vi "initialize_dcs.vi"(8 "error in (no error)":errorcluster) -> (0 "error out":errorcluster, 2 "Dust Spot Array":T1[](array[typedef]), 3 "Dust Point Array":T2[](array[typedef]))   [LabVIEW 2012]
uses:
  dcs points.ctl
  dcs_spot.ctl
  <vilib>/addons/database/Connection.llb/Conn Execute.vi
  <vilib>/addons/database/Recordset.llb/Rec Fetch Recordset Data (R).vi
  <vilib>/addons/database/Recordset.llb/Rec Destroy - Connection.vi
  <vilib>/addons/database/_DB Variant To Data/Database Variant To Data.xnode
  <vilib>/addons/database/NI_Database_API.lvlib
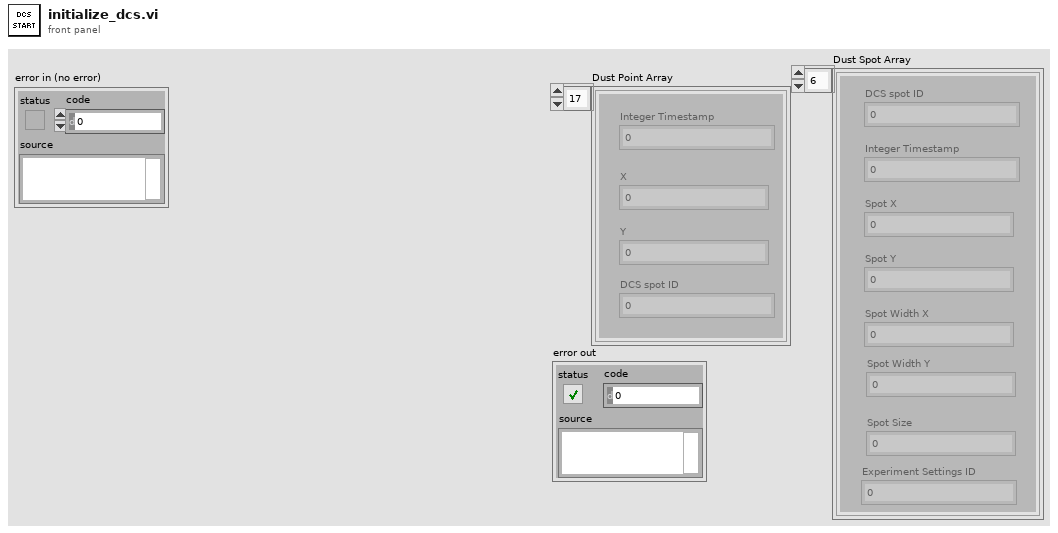
[diagram p1: front panel]
types:
  T1 = typedef "dcs_spot.ctl" = cluster{"DCS spot ID":i32, "Integer Timestamp":i64, "Spot X":dbl, "Spot Y":dbl, "Spot Width X":dbl, "Spot Width Y":dbl, "Spot Size":i32, "Experiment Settings ID":i32}
  T2 = typedef "dcs points.ctl" = cluster{"Integer Timestamp":i64, "X":dbl, "Y":dbl, "DCS spot ID":i32}
  T3 = typedef "NI_Database_API.lvlib/Conn ObjectReference.ctl" = refnum<k1>
  T4 = typedef "NI_Database_API.lvlib/Rec ObjectReference.ctl" = refnum<k1>
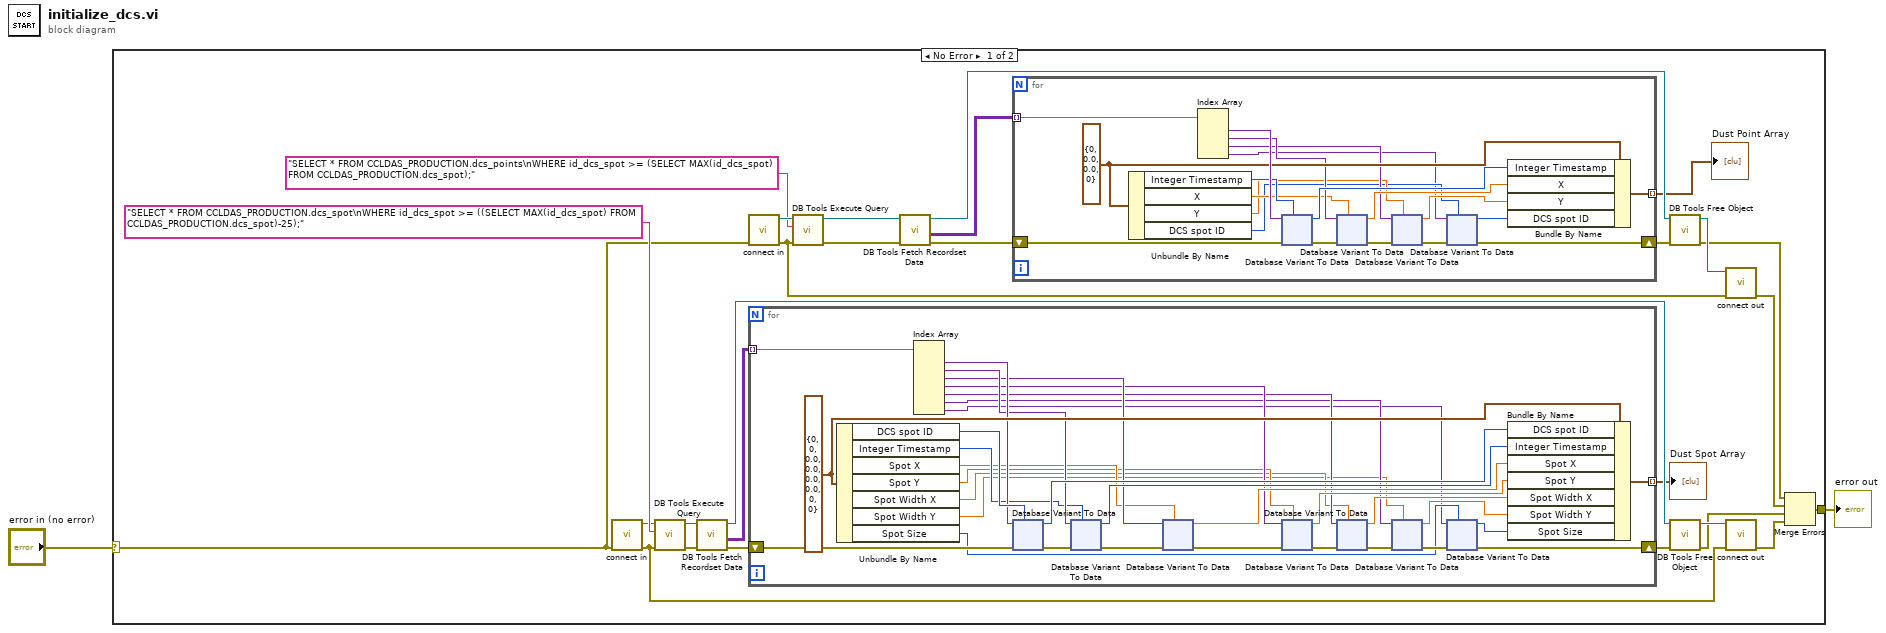
[diagram p0: block diagram]
diagram:
  n1 = case shown="No Error" "error in (no error)" {
    selector: "error in (no error)" -> [w21 w435]
    tunnel: [w3 w435] -> w1
    frame No Error {
      n2 = call "connect in.vi"("error in (no error)"=w21) -> ("error out"=w19:errorcluster, "Database Connection"=w20:T3)  [unwired: 6 in, 1 out]
      n3 = call-poly <vilib>:"DB Tools Execute Query.vi"("error in (no error)"=w19, "SQL query"="SELECT * FROM CCLDAS_PRODUCTION.dcs_spot\nWHERE id_dcs_spot >= ((SELECT MAX(id_dcs_spot) FROM CCLDAS_PRODUCTION.dcs_spot)-25);", "connection reference"=w20) -> ("error out"=w27:errorcluster, "recordset reference"=w28:T4)  [unwired: 5 in]
      n4 = call-poly <vilib>:"DB Tools Fetch Recordset Data.vi"("error in (no error)"=w27, "recordset reference"=w28) -> ("error out"=w8:errorcluster, "recordset data"=w9:variant[][], "recordset reference out"=w22:T4)  [unwired: 3 in]
      n5 = call "connect in.vi"("error in (no error)"=w21) -> ("error out"=w17:errorcluster, "Database Connection"=w26:T3)  [unwired: 6 in, 1 out]
      n6 = for {
        tunnel: w9 -> [w210] mode=indexing
        shift-right: [w182] -> w7
        shift-left: w8 -> [w207]
        tunnel: [w209] -> w4 mode=indexing
        w208 = T1 {"DCS spot ID"=0, "Integer Timestamp"=0, "Spot X"=0.0, "Spot Y"=0.0, "Spot Width X"=0.0, "Spot Width Y"=0.0, "Spot Size"=0, "Experiment Settings ID"=0} ("DCS spot")
        n7 = Unbundle By Name(w208) -> ("DCS spot ID"=w206:i32, "Integer Timestamp"=w201:i64, "Spot X"=w198:dbl, "Spot Y"=w193:dbl, "Spot Width X"=w189:dbl, "Spot Width Y"=w185:dbl, "Spot Size"=w180:i32)
        n8 = Index Array(array=w210) -> (element #1=w205:variant, element #2=w202:variant, element #3=w199:variant, element #4=w194:variant, element #5=w190:variant, element #6=w186:variant, element #7=w179:variant)  [unwired: 7 in]
        n9 = xnode "Database Variant To Data"("database variant"=w205, "error in (no error)"=w207, "type"=w206) -> ("data"=w204:i32, "error out"=w203:errorcluster)
        n10 = xnode "Database Variant To Data"("database variant"=w202, "error in (no error)"=w203, "type"=w201) -> ("data"=w200:i64, "error out"=w196:errorcluster)
        n11 = xnode "Database Variant To Data"("database variant"=w199, "error in (no error)"=w196, "type"=w198) -> ("data"=w197:dbl, "error out"=w195:errorcluster)
        n12 = xnode "Database Variant To Data"("database variant"=w194, "error in (no error)"=w195, "type"=w193) -> ("data"=w192:dbl, "error out"=w191:errorcluster)
        n13 = xnode "Database Variant To Data"("database variant"=w190, "error in (no error)"=w191, "type"=w189) -> ("data"=w188:dbl, "error out"=w187:errorcluster)
        n14 = xnode "Database Variant To Data"("database variant"=w186, "error in (no error)"=w187, "type"=w185) -> ("data"=w184:dbl, "error out"=w183:errorcluster)
        n15 = xnode "Database Variant To Data"("database variant"=w179, "error in (no error)"=w183, "type"=w180) -> ("data"=w181:i32, "error out"=w182:errorcluster)
        n16 = Bundle By Name(cluster=w208, "DCS spot ID"=w204, "Integer Timestamp"=w200, "Spot X"=w197, "Spot Y"=w192, "Spot Width X"=w188, "Spot Width Y"=w184, "Spot Size"=w181) -> (w209:T1)
      }
      "Dust Spot Array" <- w4
      n17 = call-poly <vilib>:"DB Tools Execute Query.vi"("error in (no error)"=w17, "SQL query"="SELECT * FROM CCLDAS_PRODUCTION.dcs_points\nWHERE id_dcs_spot >= (SELECT MAX(id_dcs_spot) FROM CCLDAS_PRODUCTION.dcs_spot);" ("format string"), "connection reference"=w26) -> ("error out"=w29:errorcluster, "recordset reference"=w30:T4)  [unwired: 5 in]
      n18 = call-poly <vilib>:"DB Tools Fetch Recordset Data.vi"("error in (no error)"=w29, "recordset reference"=w30) -> ("error out"=w10:errorcluster, "recordset data"=w11:variant[][], "recordset reference out"=w23:T4)  [unwired: 3 in]
      n19 = for {
        tunnel: w11 -> [w50] mode=indexing
        shift-right: [w37] -> w6
        shift-left: w10 -> [w44]
        tunnel: [w49] -> w5 mode=indexing
        w47 = T2 {"Integer Timestamp"=0, "X"=0.0, "Y"=0.0, "DCS spot ID"=0} ("DCS points")
        n20 = Unbundle By Name(w47) -> ("Integer Timestamp"=w46:i64, "X"=w41:dbl, "Y"=w35:dbl, "DCS spot ID"=w32:i32)
        n21 = Index Array(array=w50) -> (element #1=w48:variant, element #2=w42:variant, element #3=w36:variant, element #4=w31:variant)  [unwired: 4 in]
        n22 = xnode "Database Variant To Data"("database variant"=w48, "error in (no error)"=w44, "type"=w46) -> ("data"=w45:i64, "error out"=w43:errorcluster)
        n23 = xnode "Database Variant To Data"("database variant"=w42, "error in (no error)"=w43, "type"=w41) -> ("data"=w40:dbl, "error out"=w39:errorcluster)
        n24 = xnode "Database Variant To Data"("database variant"=w36, "error in (no error)"=w39, "type"=w35) -> ("data"=w34:dbl, "error out"=w38:errorcluster)
        n25 = xnode "Database Variant To Data"("database variant"=w31, "error in (no error)"=w38, "type"=w32) -> ("data"=w33:i32, "error out"=w37:errorcluster)
        n26 = Bundle By Name(cluster=w47, "Integer Timestamp"=w45, "X"=w40, "Y"=w34, "DCS spot ID"=w33) -> (w49:T2)
      }
      "Dust Point Array" <- w5
      n27 = call-poly <vilib>:"DB Tools Free Object.vi"("error in (no error)"=w6, "recordset reference"=w23) -> ("error out"=w15:errorcluster, "connection reference"=w16:T3)  [unwired: 8 in]
      n28 = call-poly <vilib>:"DB Tools Free Object.vi"("error in (no error)"=w7, "recordset reference"=w22) -> ("error out"=w13:errorcluster, "connection reference"=w18:T3)  [unwired: 8 in]
      n29 = call "connect out.vi"("error in (no error)"=w17, "connection reference"=w16) -> ("error out"=w14:errorcluster)  [unwired: 9 in]
      n30 = call "connect out.vi"("error in (no error)"=w19, "connection reference"=w18) -> ("error out"=w12:errorcluster)  [unwired: 9 in]
      n31 = Merge Errors(w15, w14, w13, w12) -> (w3:errorcluster)
    }
    frame Error {
    }
  }
  "error out" <- w1
